vi "Begin.vi"(8 "error in (no error)":errorcluster, 11 "Comp Trace Logger in":refnum<class "Comp Trace Logger.lvclass">) -> (0 "error out":errorcluster, 3 "Comp Trace Logger out":refnum<class "Comp Trace Logger.lvclass">)   [LabVIEW 2014, in "Comp Trace Logger.lvlib" / "Comp Trace Logger.lvclass"]
uses:
  Comp Trace Logger.lvclass
  Robot Actor Framework/Trace/Trace Class/Trace.lvclass
  Comp Trace Logger.lvclass/Comp Trace Logger.ctl
  Robot Actor Framework/Trace/Trace Listener Class/Trace Listener.lvclass
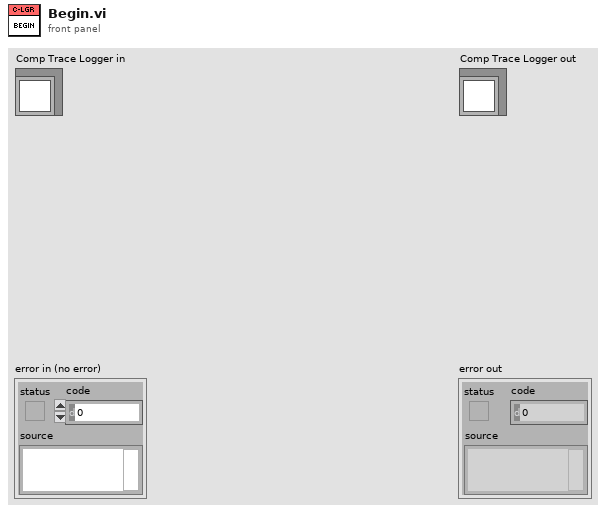
[diagram p1: front panel]
types:
  T1 = enum16{"open", "replace", "create", "open or create", "replace or create", "replace or create with confirmation"}
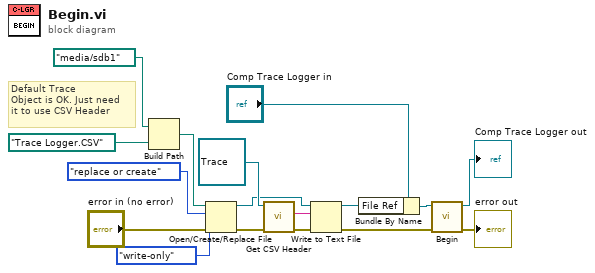
[diagram p0: block diagram]
diagram:
  # "Default Trace\nObject is OK. Just need \nit to use CSV Header"
  n1 = Build Path(base path=path "/media/sdb1" ("file path (use dialog)"), name or relative path=path "Trace Logger.CSV" ("file path (use dialog)")) -> (appended path=w12:path)
  n2 = Open/Create/Replace File(file path (use dialog)=w12, error in="error in (no error)", operation (0:open)=T1."replace or create", access (0:read/write)=enum16{"read/write", "read-only", "write-only"}."write-only") -> (refnum out=w8:refnum<file>, error out=w3:errorcluster)  [unwired: 2 in, 1 out]
  n3 = call-dynamic "Get CSV Header.vi"("error in (no error)"=w3, "Trace in"=refnum<class "Trace.lvclass"> refnum ("Robot Actor Framework.lvlib:Trace.lvlib:Trace.lvclass")) -> ("error out"=w2:errorcluster, "CSV Header"=w7:string)  [unwired: 7 in, 1 out]
  n4 = Write to Text File(file (use dialog)=w8, text=w7, error in=w2) -> (refnum out=w9:refnum<file>, error out=w4:errorcluster)  [unwired: 1 in, 1 out]
  n5 = Bundle By Name(cluster="Comp Trace Logger in", "File Ref"=w9) -> (w11:refnum<class "Comp Trace Logger.lvclass">)
  n6 = call-parent "Begin.vi"("error in (no error)"=w4, "System Actor in"=w11) -> ("error out"=→"error out":errorcluster, "System Actor out"=→"Comp Trace Logger out":refnum<class "Comp Trace Logger.lvclass">)  [unwired: 8 in]
